vi "Ejercicio 2.2.vi"() -> ()   [LabVIEW 2013]
panel:
  in  "stop 2":bool
  out "Waveform Graph":dbl[](graph)
  in  "Amplitud":dbl
  in  "Frecuencia":i32
  in  "Cantidad de muestras":i32=20
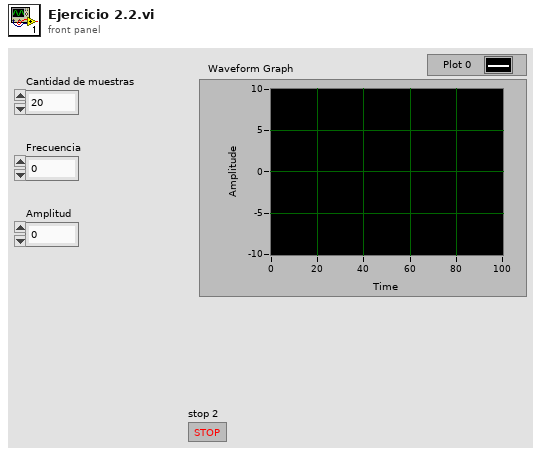
[diagram p1: front panel]
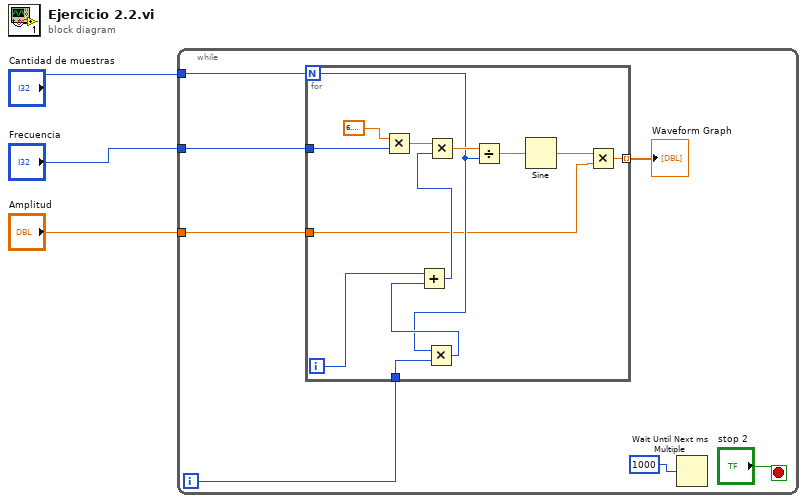
[diagram p0: block diagram]
diagram:
  n1 = while {
    tunnel: "Cantidad de muestras" -> [w7]
    tunnel: "Frecuencia" -> [w6]
    tunnel: "Amplitud" -> [w5]
    i -> [w4]
    stop <- "stop 2" stop-if-true
    n2 = for {
      N: w7 -> [w14]
      tunnel: [w18] -> w8 mode=indexing
      tunnel: w6 -> [w13]
      tunnel: w5 -> [w12]
      tunnel: w4 -> [w11]
      i -> [w17]
      n3 = Multiply(x=6.283185307179586, y=w13) -> (x*y=w23:dbl)
      n4 = Multiply(x=w14, y=w11) -> (x*y=w16:i32)
      n5 = Add(x=w17, y=w16) -> (x+y=w15:i32)
      n6 = Multiply(x=w23, y=w15) -> (x*y=w21:dbl)
      n7 = Divide(x=w21, y=w14) -> (x/y=w20:dbl)
      n8 = Sine(x=w20) -> (sin(x)=w19:dbl)
      n9 = Multiply(x=w19, y=w12) -> (x*y=w18:dbl)
    }
    "Waveform Graph" <- w8
    n10 = Wait Until Next ms Multiple(millisecond multiple=1000) -> ()  [unwired: 1 out]
  }
